vi "Init Discovery Service.vi"(8 "error in (no error)":errorcluster, 11 "Vecto in":refnum<class "Vecto.lvclass">) -> (0 "error out":errorcluster, 3 "Vecto out":refnum<class "Vecto.lvclass">)   [LabVIEW 2020, in "Vecto.lvlib" / "Vecto.lvclass"]
uses:
  Vecto.lvclass
  NodeDiscovery/NodeDiscovery.lvclass
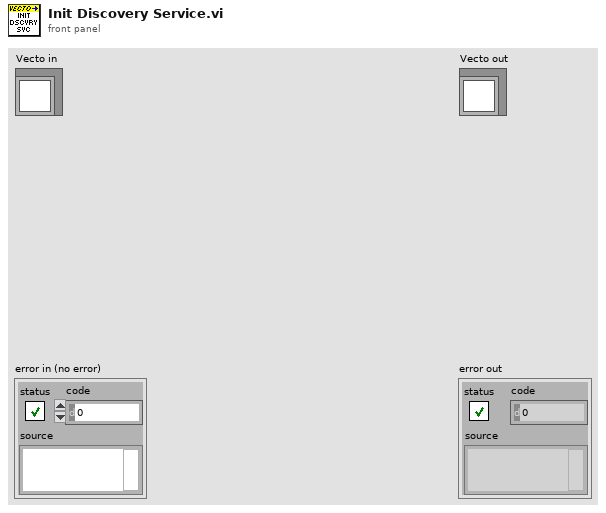
[diagram p1: front panel]
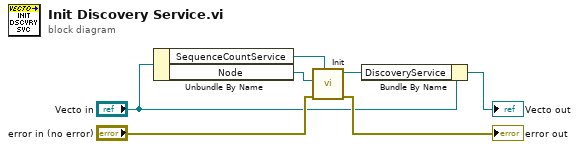
[diagram p0: block diagram]
diagram:
  n1 = Unbundle By Name("Vecto in") -> ("SequenceCountService"=w1:refnum<class "SequenceCountService.lvclass">, "Node"=w5:refnum<class "Node Config.lvclass">)
  n2 = call "Init.vi"("SequenceCountService"=w1, "error in (no error)"="error in (no error)", "Node"=w5) -> ("error out"=→"error out":errorcluster, "DiscoveryService out"=w3:refnum<class "NodeDiscovery.lvclass">)  [unwired: 7 in]
  n3 = Bundle By Name(cluster="Vecto in", "DiscoveryService"=w3) -> (→"Vecto out":refnum<class "Vecto.lvclass">)
